vi "SubVI Read Waveform File.vi"(7 "同时播放？":bool, 8 "错误输入（无错误）":errorcluster, 9 "音频输出任务ID":T1 format="%.0x", 10 "每通道采样数":i32=-1 caption="每通道采样总数（-1: 全部）", 11 "声音文件引用句柄":T2) -> (0 "错误输出":errorcluster, 1 "音频输出任务ID":T1 format="%.0x", 3 "音频数据输出":waveform(dbl), 4 "文件结束?":bool)   [LabVIEW 2015]
uses:
  <vilib>/sound2/lvsound2.llb/Sound Output Task ID.ctl
  <vilib>/sound2/lvsound2.llb/Sound File Refnum.ctl
  <vilib>/sound2/lvsound2.llb/Sound File Read (DBL).vi
  <vilib>/sound2/lvsound2.llb/Sound Output Write (DBL).vi
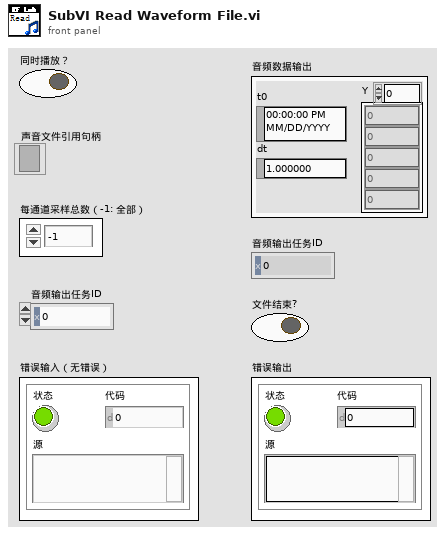
[diagram p1: front panel]
types:
  T1 = typedef "Sound Output Task ID.ctl" = u32
  T2 = typedef "Sound File Refnum.ctl" = refnum<file>
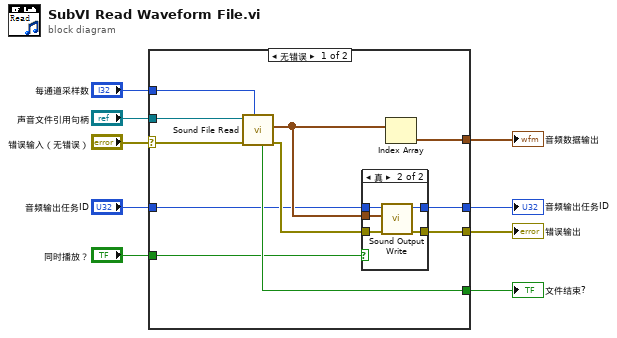
[diagram p0: block diagram]
diagram:
  n1 = case shown="无错误" "错误输入（无错误）" {
    selector: "错误输入（无错误）" -> [w10 w28]
    tunnel: [w20 w28] -> w9
    tunnel: [w18 _] -> w8
    tunnel: [w17 _] -> w7
    tunnel: [w16 _] -> w6
    tunnel: "声音文件引用句柄" -> [w15 _]
    tunnel: "音频输出任务ID" -> [w13 _]
    tunnel: "每通道采样数" -> [w12 _]
    tunnel: "同时播放？" -> [w11 _]
    frame No Error {
      n2 = call-poly <vilib>:"Sound File Read.vi"("number of samples/ch (-1: all)"=w12, "error in (no error)"=w10, "sound file refnum"=w15) -> ("error out"=w19:errorcluster, "data"=w14:waveform(dbl)[], "end of file?"=w16:bool)  [unwired: 4 in, 2 out]
      n3 = case shown="真" w11 {
        tunnel: [w21 w27] -> w20
        tunnel: w19 -> [w21 w26]
        tunnel: [w22 w25] -> w17
        tunnel: w14 -> [_ w24]
        tunnel: w13 -> [w22 w23]
        frame False {
        }
        frame True {
          n4 = call-poly <vilib>:"Sound Output Write.vi"("error in (no error)"=w26, "data"=w24, "task ID"=w23) -> ("error out"=w27:errorcluster, "task ID out"=w25:T1)  [unwired: 7 in]
        }
      }
      n5 = Index Array(array=w14) -> (element=w18:waveform(dbl))  [unwired: 1 in]
    }
    frame Error {
    }
  }
  "错误输出" <- w9
  "音频数据输出" <- w8
  "音频输出任务ID" <- w7
  "文件结束?" <- w6
